vi "setupVersion_May6.vi"() -> (3 "Keithley 6431":bool, 4 "J-KEM2":bool, 6 "Keithley 2421":bool, 8 "SRS QCM 2":bool, 10 "error IO":errorcluster, 12 "Arduino2":bool, 14 "Pressure control 2":bool, 15 "Save file path 2":path)   [LabVIEW 2014]
panel:
  in  "Save file path":path
  in  "Pressure control":bool
  in  "J-KEM":bool
  in  "Arduino":bool
  in  "Keithley 6430":bool
  in  "Keithley 2420":bool
  in  "SRS QCM":bool
  in  "OK":bool
  # "Instruments Connected"
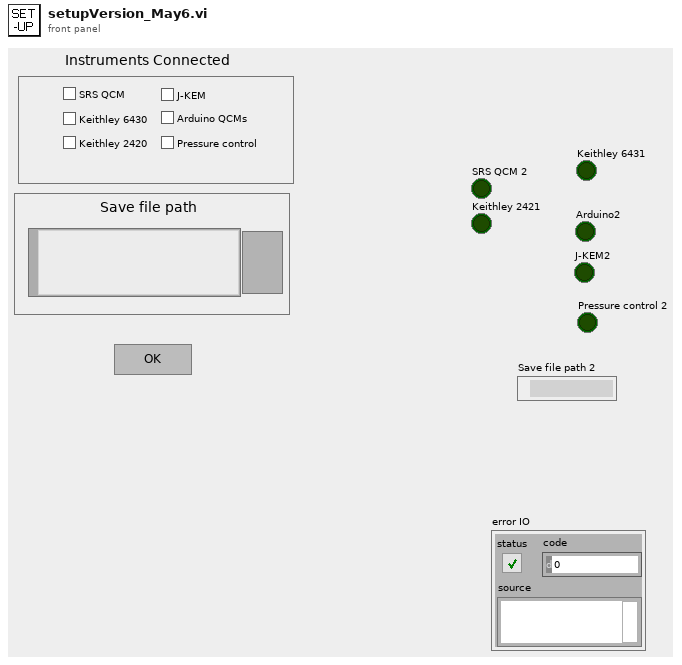
[diagram p1: front panel]
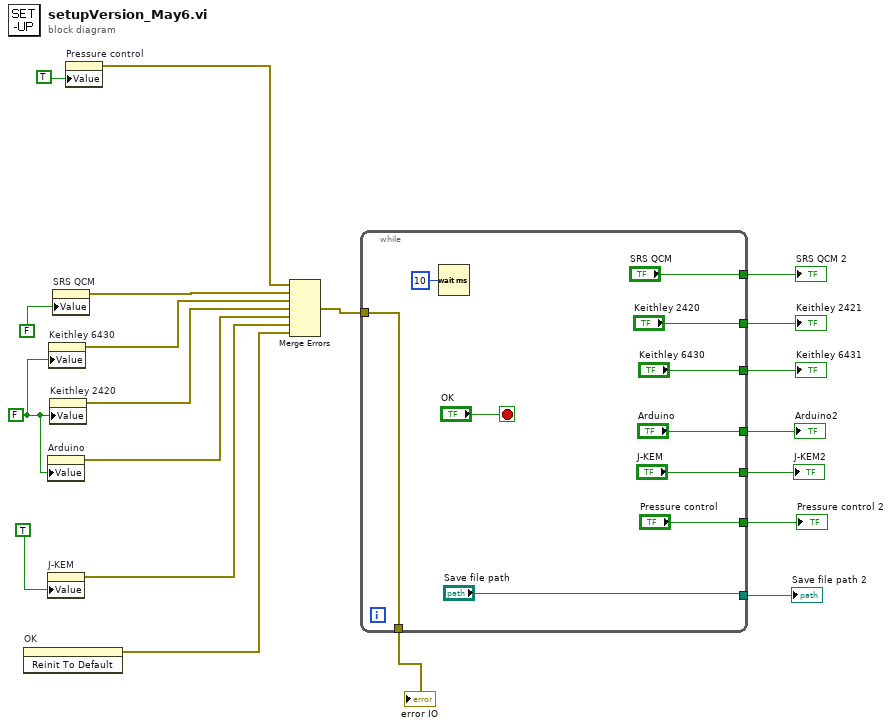
[diagram p0: block diagram]
diagram:
  w2 = FALSE ("Auto Stop")
  n1 = invoke on="OK" class="Bool" method="Reinit To Default"() -> (error out=w15:errorcluster)  [unwired: 3 in, 2 out]
  n2 = property on="Arduino" class="Bool (strict)"("Value"=w2) -> (error out=w10:errorcluster)  [unwired: 2 in, 1 out]
  n3 = property on="J-KEM" class="Bool (strict)"("Value"=TRUE ("Auto Stop")) -> (error out=w8:errorcluster)  [unwired: 2 in, 1 out]
  n4 = property on="Keithley 6430" class="Bool (strict)"("Value"=w2) -> (error out=w12:errorcluster)  [unwired: 2 in, 1 out]
  n5 = property on="Keithley 2420" class="Bool (strict)"("Value"=w2) -> (error out=w14:errorcluster)  [unwired: 2 in, 1 out]
  n6 = property on="SRS QCM" class="Bool (strict)"("Value"=FALSE ("Auto Stop")) -> (error out=w11:errorcluster)  [unwired: 2 in, 1 out]
  n7 = property on="Pressure control" class="Bool (strict)"("Value"=TRUE ("Auto Stop")) -> (error out=w1:errorcluster)  [unwired: 2 in, 1 out]
  n8 = Merge Errors(w1, w11, w12, w14, w10, w8, w15) -> (w20:errorcluster)
  n9 = while {
    tunnel: w20 -> [w21]
    tunnel: ["SRS QCM"] -> w19
    tunnel: ["Keithley 2420"] -> w18
    tunnel: ["Keithley 6430"] -> w17
    tunnel: ["Arduino"] -> w16
    tunnel: ["J-KEM"] -> w9
    tunnel: ["Pressure control"] -> w6
    tunnel: ["Save file path"] -> w5
    tunnel: [w21] -> w3
    stop <- "OK" stop-if-true
    n10 = Wait (ms)(milliseconds to wait=u32 10) -> ()  [unwired: 1 out]
  }
  "SRS QCM 2" <- w19
  "Keithley 2421" <- w18
  "Keithley 6431" <- w17
  "Arduino2" <- w16
  "J-KEM2" <- w9
  "Pressure control 2" <- w6
  "Save file path 2" <- w5
  "error IO" <- w3
